vi "Excel_Calc_Bottom_RowNum.vi"(0 "Excel._Worksheet In":refnum<k7>, 11 "error in (no error)":errorcluster) -> (4 "Excel._Worksheet Out":refnum<k7>, 14 "bottom row#":i32, 15 "error out":errorcluster)   [LabVIEW 2017, in "NI_ReportGenerationToolkit.lvlib"]
uses:
  <vilib>/addons/_office/NI_ReportGenerationToolkit.lvlib
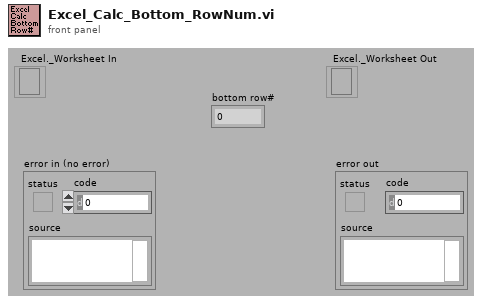
[diagram p1: front panel]
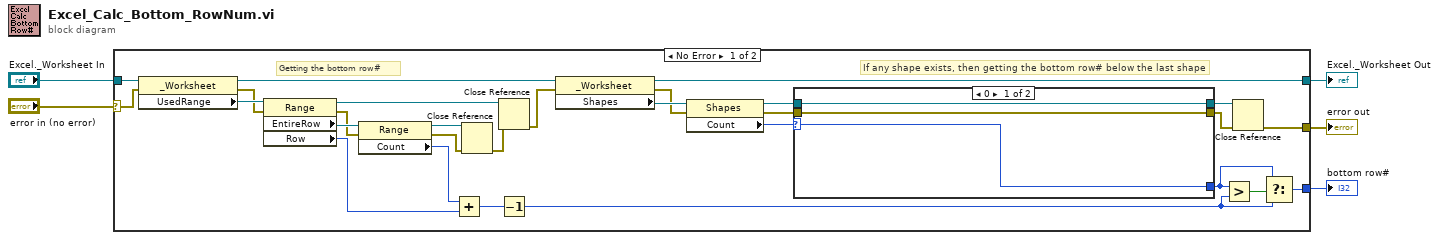
[diagram p0: block diagram]
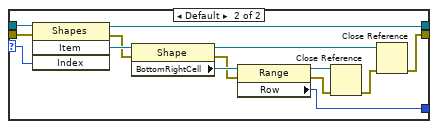
[diagram p2: hidden frame]
diagram:
  n1 = case shown="No Error" "error in (no error)" {
    selector: "error in (no error)" -> [w8 w51]
    tunnel: "Excel._Worksheet In" -> [w21 w52]
    tunnel: [w16 w52] -> w4
    tunnel: [w13 w51] -> w3
    tunnel: [w9 _] -> w2
    frame No Error {
      # "If any shape exists, then getting the bottom row# below the last shape"
      # "Getting the bottom row#"
      n2 = property class="_Worksheet"(reference=w21, error in=w8) -> (reference out=w20:refnum<k7>, error out=w31:errorcluster, "UsedRange"=w32:refnum<k7>)
      n3 = property class="Range"(reference=w32, error in=w31) -> (reference out=w24:refnum<k7>, error out=w28:errorcluster, "EntireRow"=w33:refnum<k7>, "Row"=w29:i32)
      n4 = property class="Range"(reference=w33, error in=w28) -> (reference out=w27:refnum<k7>, error out=w26:errorcluster, "Count"=w30:i32)
      n5 = Add(x=w30, y=w29) -> (x+y=w12:i32)
      n6 = Close Reference(reference=w27, error in (no error)=w26) -> (error out=w25:errorcluster)
      n7 = Close Reference(reference=w24, error in (no error)=w25) -> (error out=w19:errorcluster)
      n8 = Decrement(x=w12) -> (x-1=w10:i32)
      n9 = property class="_Worksheet"(reference=w20, error in=w19) -> (reference out=w16:refnum<k7>, error out=w17:errorcluster, "Shapes"=w18:refnum<k7>)
      n10 = property class="Shapes"(reference=w18, error in=w17) -> (reference out=w23:refnum<k7>, error out=w22:errorcluster, "Count"=w6:i32)
      n11 = case shown="0" w6 {
        selector: w6 -> [w34 w37]
        tunnel: w23 -> [w35 w42]
        tunnel: w22 -> [w36 w41]
        tunnel: [w34 w40] -> w7
        tunnel: [w36 w39] -> w14
        tunnel: [w35 w38] -> w15
        frame 0 {
        }
        frame Default {
          n12 = invoke class="Shapes" method="Item"(reference=w42, error in=w41, "Index"=w37) -> (reference out=w38:refnum<k7>, error out=w48:errorcluster, "Item"=w49:refnum<k7>)  [unwired: 1 in, 1 out]
          n13 = property class="Shape"(reference=w49, error in=w48) -> (reference out=w43:refnum<k7>, error out=w46:errorcluster, "BottomRightCell"=w47:refnum<k7>)
          n14 = property class="Range"(reference=w47, error in=w46) -> (reference out=w45:refnum<k7>, error out=w44:errorcluster, "Row"=w40:i32)
          n15 = Close Reference(reference=w45, error in (no error)=w44) -> (error out=w50:errorcluster)
          n16 = Close Reference(reference=w43, error in (no error)=w50) -> (error out=w39:errorcluster)
        }
      }
      n17 = Greater?(x=w7, y=w10) -> (0:w11:bool)
      n18 = Close Reference(reference=w15, error in (no error)=w14) -> (error out=w13:errorcluster)
      n19 = Select(t=w7, s=w11, f=w10) -> (s? t:f=w9:i32)
    }
    frame Error {
    }
  }
  "Excel._Worksheet Out" <- w4
  "bottom row#" <- w2
  "error out" <- w3
